vi "Create.vi"(7 "buffer size (10)":i32=10, 8 "error in (no error)":errorcluster, 10 "Ctrl Val.Set All":T1[](array[typedef]), 11 "name (unnamed)":string) -> (0 "error out":errorcluster, 3 "UndoObject out":refnum<class "UndoObject.lvclass">)   [LabVIEW 2015, in "UndoLibrary.lvlib" / "UndoObject.lvclass"]
doc: "This VI creates the references to store the values of the controls.\n\n- x.current: Contains the current value of the controls. (Size: 1).\n- x.undo: Allows to store the changes in the controls. (Size: Buffer).\n- x.redo: Allows to store the changes in the controls. (Size: Buffer)."
uses:
  UndoObject.lvclass
  Support VIs/DataClass/Controls/cluster_Control Value.ctl
  Support VIs/DataClass/DataObject.lvclass
  Support VIs/DataClass/DataObject.lvclass/DataObject.ctl
  UndoObject.lvclass/UndoObject.ctl
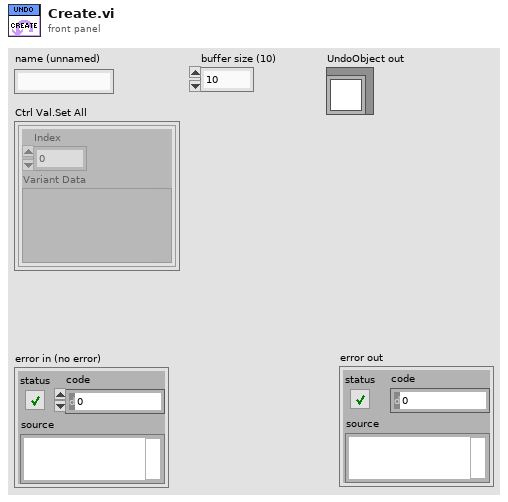
[diagram p1: front panel]
types:
  T1 = typedef "UndoLibrary.lvlib/DataObject.lvclass/cluster_Control Value.ctl" = cluster{"Index":i32, "Variant Data":variant}
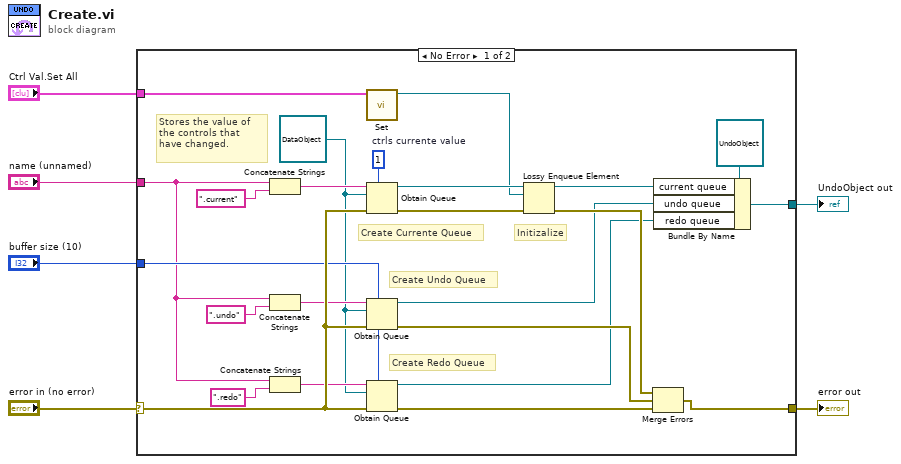
[diagram p0: block diagram]
diagram:
  n1 = case shown="No Error" "error in (no error)" {
    selector: "error in (no error)" -> [w28 w31]
    tunnel: "Ctrl Val.Set All" -> [w12 _]
    tunnel: "buffer size (10)" -> [w26 _]
    tunnel: "name (unnamed)" -> [w24 _]
    tunnel: [w13 _] -> w1
    tunnel: [w17 w31] -> w2
    frame No Error {
      w10 = refnum<class "DataObject.lvclass"> refnum ("UndoLibrary.lvlib:DataObject.lvclass")
      w27 = 1  # ctrls currente value
      # "Stores the value of the controls that have changed."
      # "Create Redo Queue"
      # "Create Undo Queue"
      # "Initizalize"
      # "Create Currente Queue"
      n2 = Concatenate Strings(w24, ".current" ("name (unnamed)")) -> (w20:string)
      n3 = Concatenate Strings(w24, ".undo" ("name (unnamed)")) -> (w19:string)
      n4 = Concatenate Strings(w24, ".redo" ("name (unnamed)")) -> (w18:string)
      n5 = call "Set.vi"("Conrol Value[]"=w12) -> ("DataObject out"=w11:refnum<class "DataObject.lvclass">)  [unwired: 9 in, 1 out]
      n6 = Obtain Queue(max queue size (-1, unlimited)=w27, name (unnamed)=w20, element data type=w10, error in (no error)=w28) -> (queue out=w29:refnum<queue>, error out=w30:errorcluster)  [unwired: 1 in, 1 out]
      n7 = Obtain Queue(max queue size (-1, unlimited)=w26, name (unnamed)=w19, element data type=w10, error in (no error)=w28) -> (queue out=w8:refnum<queue>, error out=w15:errorcluster)  [unwired: 1 in, 1 out]
      n8 = Obtain Queue(max queue size (-1, unlimited)=w26, name (unnamed)=w18, element data type=w10, error in (no error)=w28) -> (queue out=w7:refnum<queue>, error out=w25:errorcluster)  [unwired: 1 in, 1 out]
      n9 = Lossy Enqueue Element(queue=w29, element=w11, error in (no error)=w30) -> (queue out=w9:refnum<queue>, error out=w16:errorcluster)  [unwired: 2 out]
      n10 = Merge Errors(w16, w15, w25) -> (w17:errorcluster)
      n11 = Bundle By Name(cluster=refnum<class "UndoObject.lvclass"> refnum ("UndoLibrary.lvlib:UndoObject.lvclass"), "current queue"=w9, "undo queue"=w8, "redo queue"=w7) -> (w13:refnum<class "UndoObject.lvclass">)
    }
    frame Error {
    }
  }
  "error out" <- w2
  "UndoObject out" <- w1
